vi "Configure Serial Port.vi"(5 "Timeout":u32=10000, 6 "Flow Control":u16(ring) items=["None", "XON/XOFF", "RTS/CTS", "XON/XOFF & RTS/CTS", "DTR/DSR", "XON/XOFF & DTR/DSR"], 7 "data bits":u16, 8 "error in (no error)":errorcluster, 9 "Parity":u16(ring)=2 items=["None", "Odd", "Even", "Mark", "Space"], 10 "Baud Rate":u32=9600, 11 "VISA Refnum in":refnum<visa-resource-name>) -> (0 "error out":errorcluster)   [LabVIEW 2015, in "Modbus Library.lvlib" / "Serial Shared Components.lvlib"]
doc: "Configures a selected serial port with various options."
uses:
  Serial Shared Components.lvlib
  <vilib>/Instr/_visa.llb/VISA Flush IO Buffer Mask.ctl
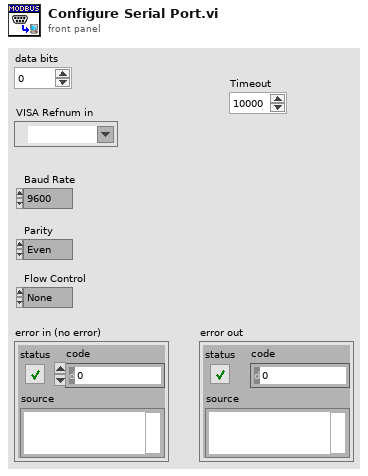
[diagram p1: front panel]
types:
  T1 = typedef "VISA Flush IO Buffer Mask.ctl" = u16
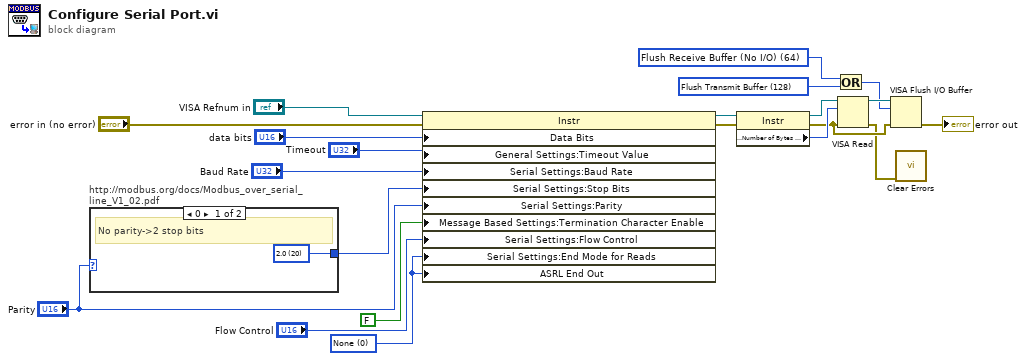
[diagram p0: block diagram]
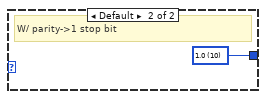
[diagram p2: hidden frame]
diagram:
  w9 = T1 128 items=["Flush Receive Buffer"=16, "Write Transmit Buffer to Device"=32, "Flush Receive Buffer (No I/O)"=64, "Flush Transmit Buffer"=128] ("Mask")
  w8 = T1 64 items=["Flush Receive Buffer"=16, "Write Transmit Buffer to Device"=32, "Flush Receive Buffer (No I/O)"=64, "Flush Transmit Buffer"=128] ("Mask")
  w1 = u16 0 items=["None", "LastBit", "TermChar"] ("Serial Settings:Serial End Mode for Reads")
  n1 = case "http://modbus.org/docs/Modbus_over_serial_line_V1_02.pdf" shown="0" "Parity" {
    tunnel: [w22 w23] -> w6
    frame 0 {
      w22 = u16 20 items=["1.0"=10, "1.5"=15, "2.0"=20] ("Serial Settings:Serial Stop Bits")
      # "No parity->2 stop bits"
    }
    frame Default {
      w23 = u16 10 items=["1.0"=10, "1.5"=15, "2.0"=20] ("Serial Settings:Serial Stop Bits")
      # "W/ parity->1 stop bit"
    }
  }
  n2 = property class="Instr"(reference="VISA Refnum in", error in="error in (no error)", "Data Bits"="data bits", "General Settings:Timeout Value"="Timeout", "Serial Settings:Baud Rate"="Baud Rate", "Serial Settings:Stop Bits"=w6, "Serial Settings:Parity"="Parity", "Message Based Settings:Termination Character Enable"=FALSE, "Serial Settings:Flow Control"="Flow Control", "Serial Settings:End Mode for Reads"=w1, "ASRL End Out"=w1) -> (reference out=w14:refnum<visa-resource-name>, error out=w13:errorcluster)
  n3 = property class="Instr"(reference=w14, error in=w13) -> (reference out=w16:refnum<visa-resource-name>, error out=w3:errorcluster, "Serial Settings:Number of Bytes at Serial Port"=w17:u32)
  n4 = Or(x=w8, y=w9) -> (x .or. y?=w7:T1)
  n5 = VISA Read(VISA resource name=w16, byte count=w17, error in (no error)=w3) -> (VISA resource name out=w15:refnum<visa-resource-name>, error out=w2:errorcluster)  [unwired: 2 out]
  n6 = VISA Flush I/O Buffer(VISA resource name=w15, mask (16)=w7, error in (no error)=w3) -> (error out=→"error out":errorcluster)  [unwired: 1 out]
  n7 = call <vilib>:"Clear Errors.vi"("error in (no error)"=w2) -> ()  [unwired: 5 in, 2 out]
